vi "updateQtn.vi"(0 "reference in":refnum<class "Items Controller.lvclass">, 5 "dataIN":string[](array[string]), 7 "storageIN":string[][](array[string]), 9 "IN-OUT":bool, 11 "error in (no error)":errorcluster) -> (4 "reference out":refnum<class "Items Controller.lvclass">, 8 "S/N":string, 10 "storageOUT":string[][](array[string]), 15 "error out":errorcluster)   [LabVIEW 2016, in "Items Controller.lvclass"]
uses:
  Items Controller.lvclass
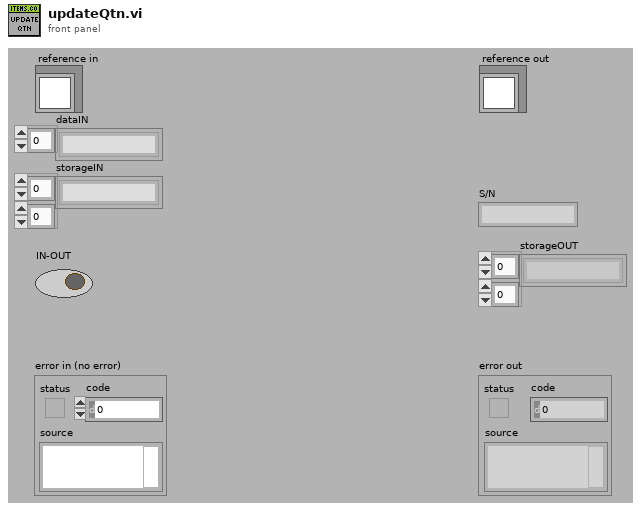
[diagram p1: front panel]
types:
  T1 = typedef "Items Controller.lvclass/ObjectAttributesRef.ctl" = refnum<data-value>
  T2 = typedef "Items Controller.lvclass/ObjectAttributes.ctl" = cluster{"MyAttribute":dbl, "data":string[][][], "file_controller_ref":refnum<class "File Controller.lvclass">, "checkIN_ref":refnum<class "checkIN.lvclass">, "checkOUT_ref":refnum<class "checkOUT.lvclass">, "item_ref":refnum<class "item.lvclass">}
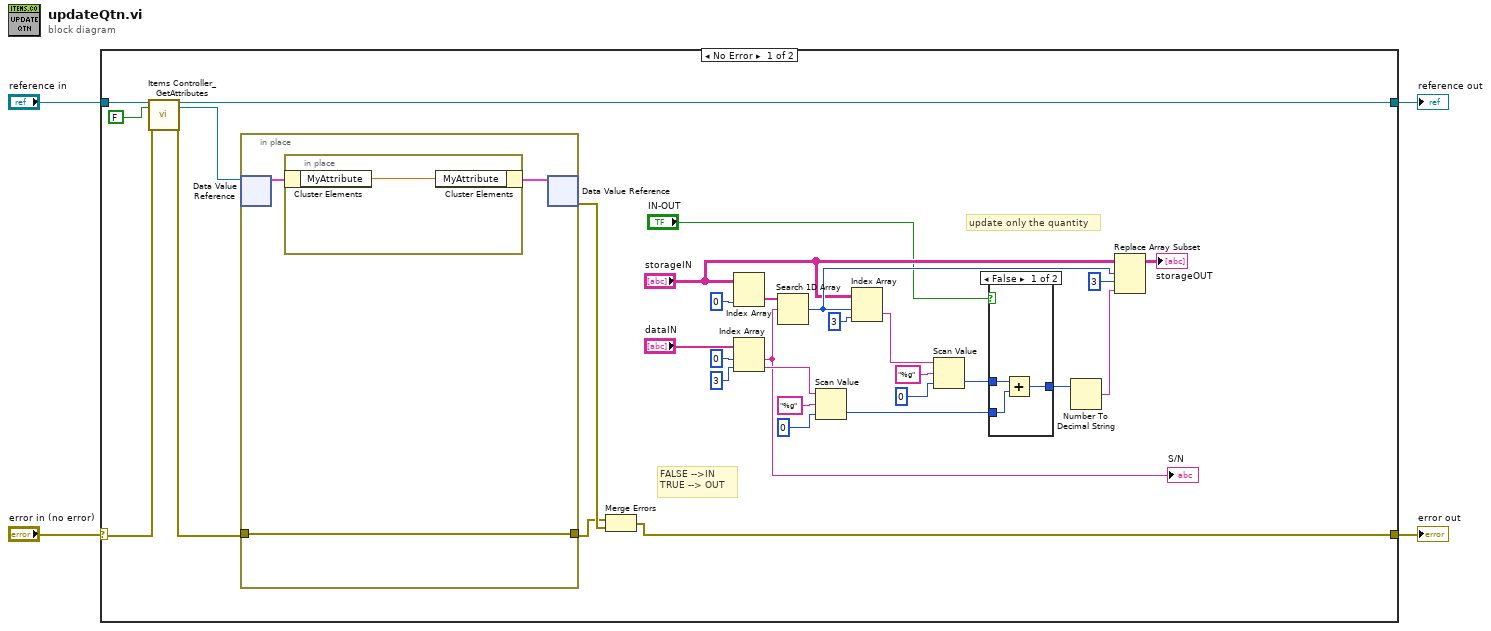
[diagram p0: block diagram]
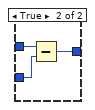
[diagram p2: hidden frame]
diagram:
  n1 = case shown="No Error" "error in (no error)" {
    selector: "error in (no error)" -> [w31 w47]
    tunnel: [w27 w47] -> w3
    tunnel: [w29 w46] -> w1
    tunnel: "reference in" -> [w33 w46]
    frame No Error {
      # "FALSE -->IN\nTRUE --> OUT"
      # "update only the quantity"
      n2 = call "Items Controller_GetAttributes.vi"("reference in"=w33, "return data? (T)"=FALSE, "error in (no error)"=w31) -> ("reference out"=w29:refnum<class "Items Controller.lvclass">, "attributes ref"=w28:T1, "error out"=w30:errorcluster)  [unwired: 13 in, 1 out]
      n3 = in-place {
        in-place-border: w30 -> [w42]
        in-place-border: [w42] -> w34
        n4 = in-place-dvr #1(w28) -> (w43:T2)  [unwired: 1 out]
        n5 = in-place {
          n6 = in-place-cluster #2(w43) -> ("MyAttribute"=w45:dbl)
          n7 = in-place-cluster #2("MyAttribute"=w45) -> (w44:T2)
        }
        n8 = in-place-dvr #1(w44) -> (w35:errorcluster)  [unwired: 1 out]
      }
      n9 = Merge Errors(w34, w35) -> (w27:errorcluster)
      n10 = Index Array(array="storageIN", index (col)=0 ("index")) -> (element=w25:string[])  [unwired: 1 in]
      n11 = Index Array(array="dataIN", index #1=0 ("index"), index #2=3 ("index")) -> (element #1=w18:string, element #2=w23:string)
      "S/N" <- w18
      n12 = Search 1D Array(1D array=w25, element=w18) -> (index of element=w22:i32)  [unwired: 1 in]
      n13 = Scan Value(string=w23, format string="%g", default (0 dbl)=0 ("y")) -> (value=w8:i32)  [unwired: 1 out]
      n14 = Index Array(array="storageIN", index (row)=w22, index (col)=3 ("disabled index (col)")) -> (element=w14:string)
      n15 = Scan Value(string=w14, format string="%g", default (0 dbl)=0 ("y")) -> (value=w9:i32)  [unwired: 1 out]
      n16 = case shown="False" "IN-OUT" {
        tunnel: w9 -> [w37 w41]
        tunnel: w8 -> [w38 w40]
        tunnel: [w36 w39] -> w6
        frame False {
          n17 = Add(x=w37, y=w38) -> (x+y=w36:i32)
        }
        frame True {
          n18 = Subtract(x=w41, y=w40) -> (x-y=w39:i32)
        }
      }
      n19 = Number To Decimal String(number=w6) -> (decimal integer string=w5:string)  [unwired: 1 in]
      n20 = Replace Array Subset(array="storageIN", new element=w5, index (row)=w22, index (col)=3 ("disabled index (col)")) -> (→"storageOUT":string[][])
    }
    frame Error {
    }
  }
  "error out" <- w3
  "reference out" <- w1
